vi "Resize image and strings.vi"(0 "Tab details":T2, 1 "Image label":refnum<vi>, 5 "Image position and resize":T1, 7 "Type of label":u16(ring) items=["Combo", "String"], 9 "TL":refnum<vi>, 11 "error in (no error)":errorcluster, 12 "Img Refnum":refnum<vi>) -> (15 "error out":errorcluster)   [LabVIEW 2019, in "ZenGage v3.0 UI.lvclass"]
uses:
  ZenGage v3.0 UI.lvclass
panel:
  # "e"
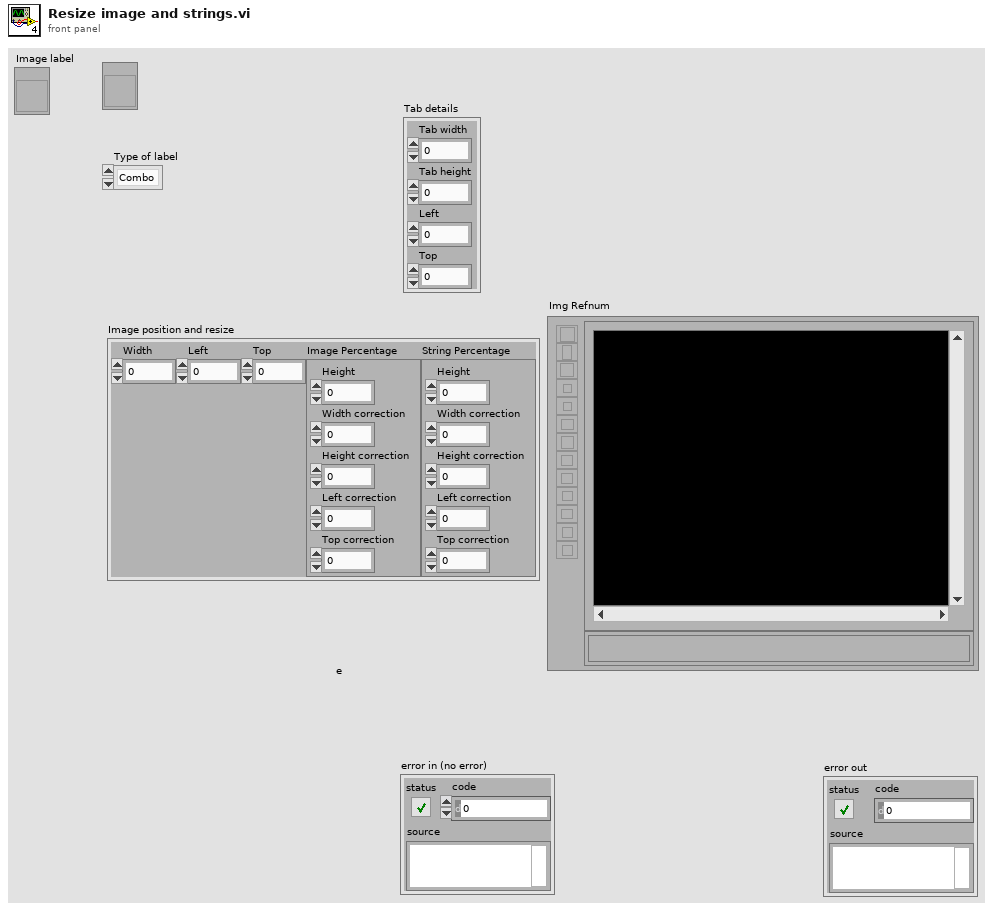
[diagram p1: front panel]
types:
  T1 = cluster{"Width":dbl, "Left":dbl, "Top":dbl, "Image Percentage":cluster{"Height":dbl, "Width correction":dbl, "Height correction":dbl, "Left correction":dbl, "Top correction":dbl}, "String Percentage":cluster{"Height":dbl, "Width correction":dbl, "Height correction":dbl, "Left correction":dbl, "Top correction":dbl}}
  T2 = cluster{"Tab width":u32, "Tab height":u32, "Left":i32, "Top":i32}
  T3 = cluster{"Height":dbl, "Width correction":dbl, "Height correction":dbl, "Left correction":dbl, "Top correction":dbl}
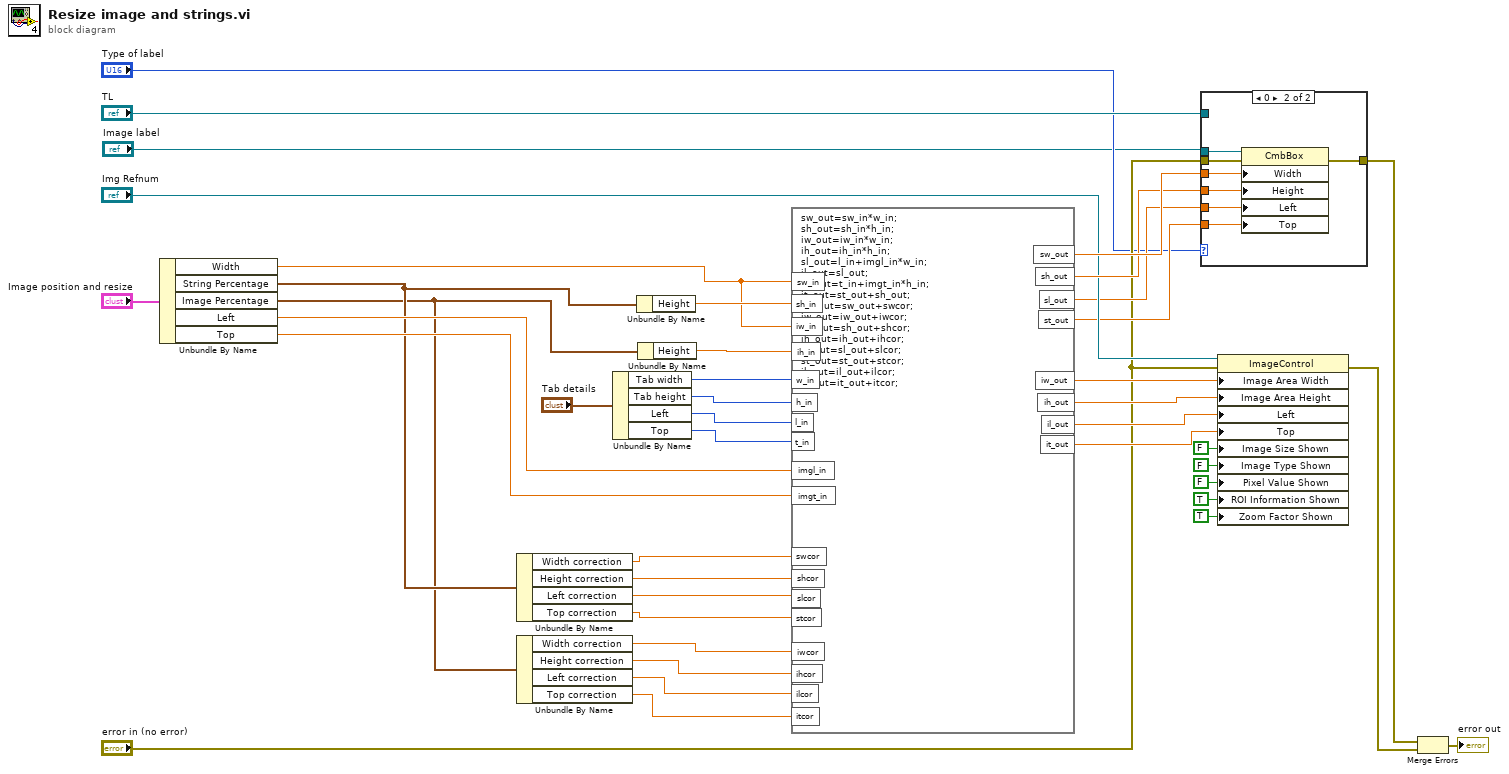
[diagram p0: block diagram]
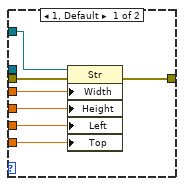
[diagram p2: hidden frame]
diagram:
  n1 = Unbundle By Name("Image position and resize") -> ("Width"=w14:dbl, "String Percentage"=w21:T3, "Image Percentage"=w20:T3, "Left"=w23:dbl, "Top"=w22:dbl)
  n2 = Unbundle By Name(w21) -> ("Width correction"=w19:dbl, "Height correction"=w18:dbl, "Left correction"=w13:dbl, "Top correction"=w12:dbl)
  n3 = Unbundle By Name(w20) -> ("Width correction"=w17:dbl, "Height correction"=w16:dbl, "Left correction"=w11:dbl, "Top correction"=w10:dbl)
  n4 = Unbundle By Name("Tab details") -> ("Tab width"=w31:u32, "Tab height"=w30:u32, "Left"=w29:i32, "Top"=w28:i32)
  n5 = Unbundle By Name(w21) -> ("Height"=w42:dbl)
  n6 = Unbundle By Name(w20) -> ("Height"=w41:dbl)
  n7 = formula code="sw_out=sw_in*w_in;\nsh_out=sh_in*h_in;\niw_out=iw_in*w_in;\nih_out=ih_in*h_in;\nsl_out=l_in+imgl_in*w_in;\nil_out=sl_out;\nst_out=t_in+imgt_in*h_in;\nit_out=st_out+sh_out;\nsw_out=sw_out+swcor;\niw_out=iw_out+iwcor;\nsh_out=sh_out+shcor;\nih_out=ih_out+ihcor;\nsl_out=sl_out+slcor;\nst_out=st_out+stcor;\nil_out=il_out+ilcor;\nit_out=it_out+itcor;"("sw_in"=w14, "sh_in"=w42, "iw_in"=w14, "ih_in"=w41, "w_in"=w31, "h_in"=w30, "l_in"=w29, "t_in"=w28, "imgl_in"=w23, "imgt_in"=w22, "swcor"=w19, "shcor"=w18, "iwcor"=w17, "ihcor"=w16, "slcor"=w13, "stcor"=w12, "ilcor"=w11, "itcor"=w10) -> ("sw_out"=w40:dbl, "sh_out"=w39:dbl, "iw_out"=w38:dbl, "ih_out"=w37:dbl, "sl_out"=w25:dbl, "st_out"=w24:dbl, "il_out"=w27:dbl, "it_out"=w26:dbl)
  n8 = case shown="0" "Type of label" {
    tunnel: w40 -> [w47 w56]
    tunnel: w39 -> [w46 w55]
    tunnel: [w49 w54] -> w35
    tunnel: "Image label" -> [_ w53]
    tunnel: w25 -> [w45 w52]
    tunnel: w24 -> [w44 w51]
    tunnel: "error in (no error)" -> [w48 w50]
    tunnel: "TL" -> [w43 _]
    frame 1, Default {
      n9 = property class="Str"(reference=w43, error in=w48, "Width"=w47, "Height"=w46, "Left"=w45, "Top"=w44) -> (error out=w49:errorcluster)  [unwired: 1 out]
    }
    frame 0 {
      n10 = property class="CmbBox"(reference=w53, error in=w50, "Width"=w56, "Height"=w55, "Left"=w52, "Top"=w51) -> (error out=w54:errorcluster)  [unwired: 1 out]
    }
  }
  n11 = property class="ImageControl"(reference="Img Refnum", error in="error in (no error)", "Image Area Width"=w38, "Image Area Height"=w37, "Left"=w27, "Top"=w26, "Image Size Shown"=FALSE ("Image Information Shown:Image Size Shown"), "Image Type Shown"=FALSE ("Image Information Shown:Image Type Shown"), "Pixel Value Shown"=FALSE ("Image Information Shown:Pixel Value Shown"), "ROI Information Shown"=TRUE ("Image Information Shown:ROI Information Shown"), "Zoom Factor Shown"=TRUE ("Image Information Shown:Zoom Factor Shown")) -> (error out=w36:errorcluster)  [unwired: 1 out]
  n12 = Merge Errors(w35, w36) -> (→"error out":errorcluster)
